vi "DAQmx Timing (Change Detection).vi"(0 "task/channels in":refnum<k21>, 1 "sample mode":i32(ring)=10178 items=["Finite Samples"=10178, "Continuous Samples"=10123, "Hardware Timed Single Point"=12522], 2 "samples per channel":i32=1000, 7 "rising edge physical channels":tag, 9 "falling edge physical channels":tag, 11 "error in":errorcluster) -> (4 "task out":refnum<k21>, 15 "error out":errorcluster)   [LabVIEW 2020]
doc: "Configures the task to acquire samples on the rising and/or falling edges of the lines or ports you specify. To detect both rising and falling edges on a line or port, wire the name of that line or port to both <B>rising edge physical channels</B> and <B>falling edge physical channels</B>."
uses:
  nilvaiu.dll
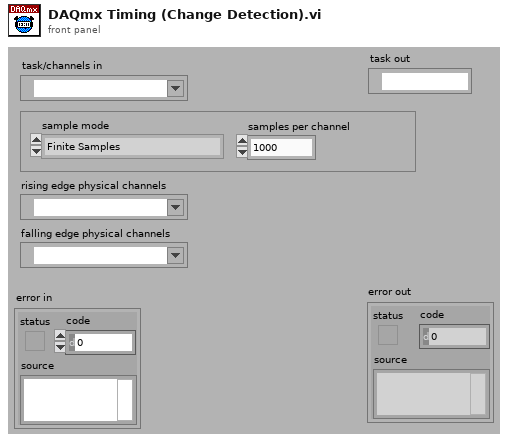
[diagram p1: front panel]
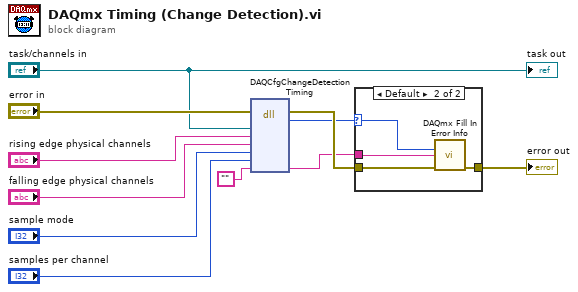
[diagram p0: block diagram]
diagram:
  n1 = dll-call lib="nilvaiu.*" fn="DAQCfgChangeDetectionTiming"(error in="error in", "taskID"="task/channels in", "risingEdgeChan"="rising edge physical channels", "fallingEdgeChan"="falling edge physical channels", "sampleMode"="sample mode", "samplesPerChannel"="samples per channel", "extendedErrorInfo"="") -> (error out=w8:errorcluster, "return type"=w6:i32, "extendedErrorInfo"=w7:string)  [unwired: 4 in, 4 out]
  n2 = case shown="Default" w6 {
    selector: w6 -> [_ w14]
    tunnel: w8 -> [w12 w16]
    tunnel: [w12 w15] -> w10
    tunnel: w7 -> [_ w13]
    frame 0 {
    }
    frame Default {
      n3 = call "DAQmx Fill In Error Info.vi"("status code"=w14, "extended error info"=w13, "error in"=w16) -> ("error out"=w15:errorcluster)  [unwired: 1 in, 11 out]
    }
  }
  "error out" <- w10
  "task out" <- "task/channels in"
